vi "niMmWave_Reciever_Create.vi"(8 "error in (no error)":errorcluster, 11 "reference in":refnum<class "niMmWave_Reciever.lvclass">) -> (0 "error out":errorcluster, 3 "reference out":refnum<class "niMmWave_Reciever.lvclass">)   [LabVIEW 2019, in "niMmWave_Reciever.lvclass"]
doc: "Constructor."
uses:
  niMmWave_Reciever.lvclass
  C:/Program Files/National Instruments/LabVIEW 2019/vi.lib/addons/_AddQ/G#Object/G#Object.lvclass
  C:/Barkhausen mmWave radar/Development/LV/Barkhausen mmWave hardware control/Host/SubVIs/mmWave instrument_class/mmWave instrument.lvclass
  <vilib>/addons/_AddQ/G#Object/G#Object.lvclass
  mmWave instrument_class/mmWave instrument.lvclass
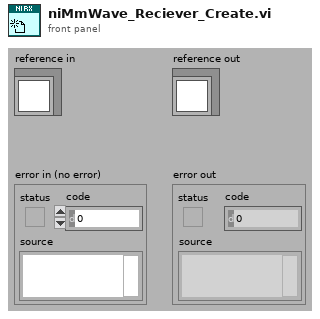
[diagram p1: front panel]
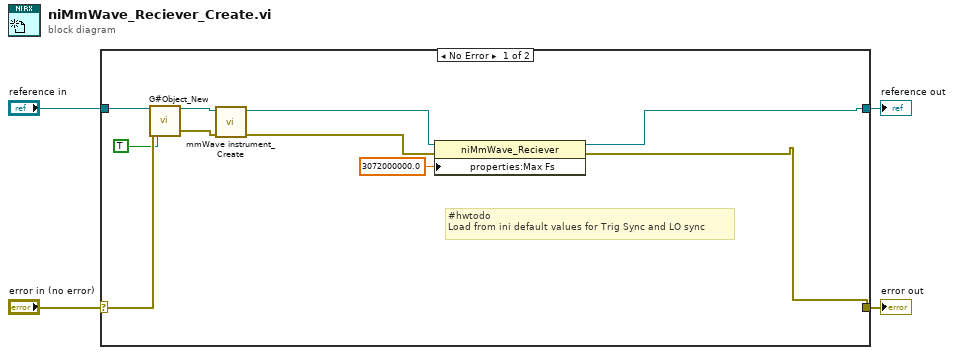
[diagram p0: block diagram]
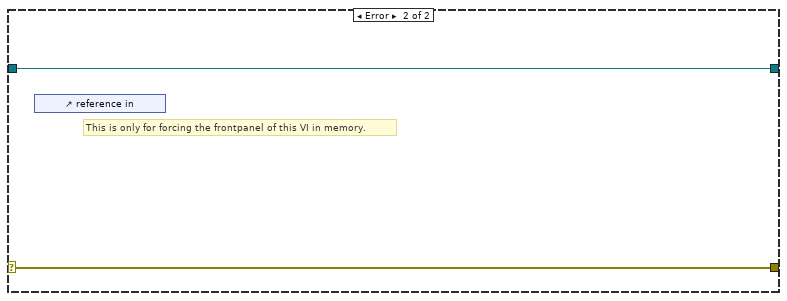
[diagram p2: hidden frame]
diagram:
  n1 = case shown="No Error" "error in (no error)" {
    selector: "error in (no error)" -> [w13 w16]
    tunnel: [w5 w16] -> w3
    tunnel: [w6 w15] -> w1
    tunnel: "reference in" -> [w14 w15]
    frame No Error {
      # "#hwtodo\nLoad from ini default values for Trig Sync and LO sync"
      n2 = call <vilib>:"G#Object_New.vi"("reference in"=w14, "error in (no error)"=w13, "user counter (T)?"=TRUE ("User Counter")) -> ("reference out"=w10:refnum<class "niMmWave_Reciever.lvclass">, "error out"=w9:errorcluster)  [unwired: 14 in, 1 out]
      n3 = call "mmWave instrument_Create.vi"("error in (no error)"=w9, "reference in"=w10) -> ("error out"=w8:errorcluster, "reference out"=w7:refnum<class "niMmWave_Reciever.lvclass">)  [unwired: 8 in]
      n4 = property class="niMmWave_Reciever"(reference=w7, error in=w8, "properties:Max Fs"=3072000000.0 ("Max Fs")) -> (reference out=w6:refnum<class "niMmWave_Reciever.lvclass">, error out=w5:errorcluster)
    }
    frame Error {
      # "This is only for forcing the frontpanel of this VI in memory."
      n5 = control-ref of="reference in"() -> ()  [unwired: 1 out]
    }
  }
  "error out" <- w3
  "reference out" <- w1
